vi "DestroyPublicEvents.vi"(8 "error in (no error)":errorcluster, 11 "Device":refnum<class "Device.lvclass">) -> (0 "error out":errorcluster, 3 "Device out":refnum<class "Device.lvclass">)   [LabVIEW 2017, in "Device.lvclass"]
doc: "JKI State Machine Objects (SMO) 1.3.0.56\nJKI - JKI\nCopyright (c) 2017, JKI"
uses:
  Device.lvclass
  <vilib>/JKI/JKI SMO/SMO/SMO.lvclass
panel:
  # "For instructions on how to use the JKI State Machine Objects, examples and video tutorials, visit:\nhttp://jki.net/state-machine-objects/\n\nJKI State Machine Objects™\nhttp://jki.net/state-machine-objects/\nCopyright (C) 2005-2015, JKI <info@jki.net>\nALL RIGHTS RESERVED"
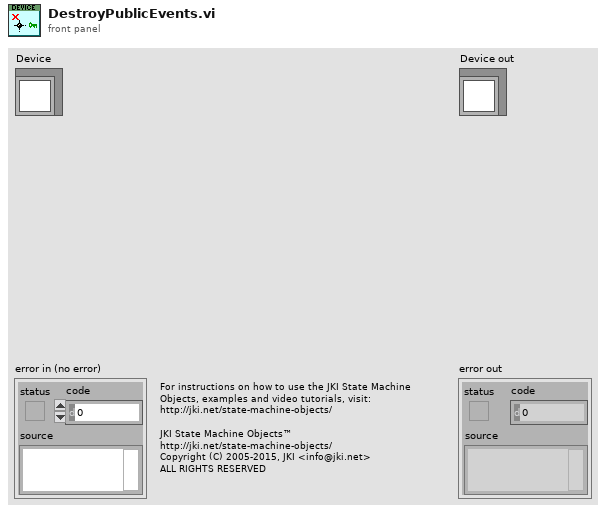
[diagram p1: front panel]
types:
  T1 = typedef "Device.lvclass/PublicEvents--Cluster.ctl" = cluster{"Initialized":refnum<user-event>, "Uninitialized":refnum<user-event>}
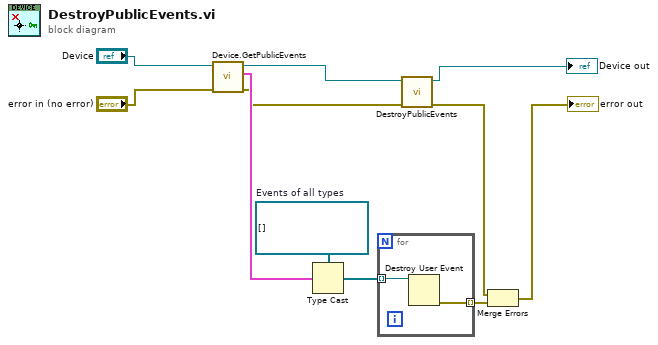
[diagram p0: block diagram]
diagram:
  w8 = refnum<user-event>[] []  # Events of all types
  n1 = call "Device.GetPublicEvents.vi"("error in (no error)"="error in (no error)", "Device in"="Device") -> ("error out"=w4:errorcluster, "Public Events"=w6:T1, "Device out"=w5:refnum<class "Device.lvclass">)  [unwired: 7 in]
  n2 = Type Cast(type=w8, x=w6) -> (*(type *) &x=w9:refnum<user-event>[])
  n3 = for {
    tunnel: w9 -> [w13] mode=indexing
    tunnel: [w12] -> w7 mode=indexing
    n4 = Destroy User Event(user event=w13) -> (error out=w12:errorcluster)  [unwired: 1 in]
  }
  n5 = call-parent "DestroyPublicEvents.vi"("error in (no error)"=w4, "SMO"=w5) -> ("error out"=w2:errorcluster, "SMO out"=→"Device out":refnum<class "Device.lvclass">)  [unwired: 8 in]
  n6 = Merge Errors(w2, w7) -> (→"error out":errorcluster)
